vi "Wyznaczenie odległości robota od sartu na podstawie współrzędnych.vi"(7 "Azymut robota\n pocz/nowy":dbl caption="Azymut robota pocz/nowy" min=0.0 max=360.0, 10 "Parametry odwzorowania Ziemi (WGS84)":cluster{"a":dbl, "b":dbl}={"a"=6378137.0, "b"=6356752.3142} {"b" format="%#.6g"; "a" format="%#.6g"}, 11 "Pocz. poł.":T1 {"UTM"."N [m]" format="%#_10g"}) -> (0 "error out":errorcluster, 2 "Rzeczywista odległość robota od startu [m]":cluster{"X [m]":dbl, "Y [m]":dbl}, 3 "Aktualne położenie":T2 {"Szerokośc geograficzna - GPS" format="%_9f"; "Długość geograficzna - GPS" format="%_9f"; "Położenie \nrobota  UTM"."E [m]" format="%#_10g"; "Położenie \nrobota  UTM"."N [m]" format="%#_12g"})   [LabVIEW 2015, in "Biblioteka moduł map v3.lvlib" / "Pomocnicze.lvlib"]
doc: "Zadaniem pliku jest wyznaczenie odległości robota od punktu startowego na podstawie znanych współrzędnych geograficznych pliku startowego oraz odczytów z odbiornika GPS."
uses:
  Pomocnicze.lvlib
  Matematyczne/Matematyczne.lvlib
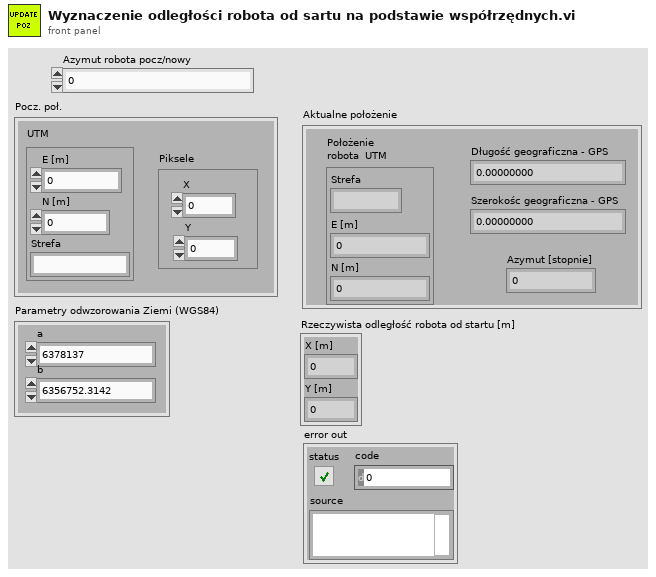
[diagram p1: front panel]
types:
  T1 = cluster{"UTM":cluster{"E [m]":dbl, "N [m]":dbl, "Strefa":string}, "Piksele":cluster{"X":i32, "Y":i32}}
  T2 = cluster{"Położenie \nrobota  UTM":cluster{"E [m]":ext, "N [m]":ext, "Strefa":string}, "Długość geograficzna - GPS":dbl, "Szerokośc geograficzna - GPS":dbl, "Azymut [stopnie]":dbl}
  T3 = cluster{"E [m]":ext, "N [m]":ext, "Strefa":string}
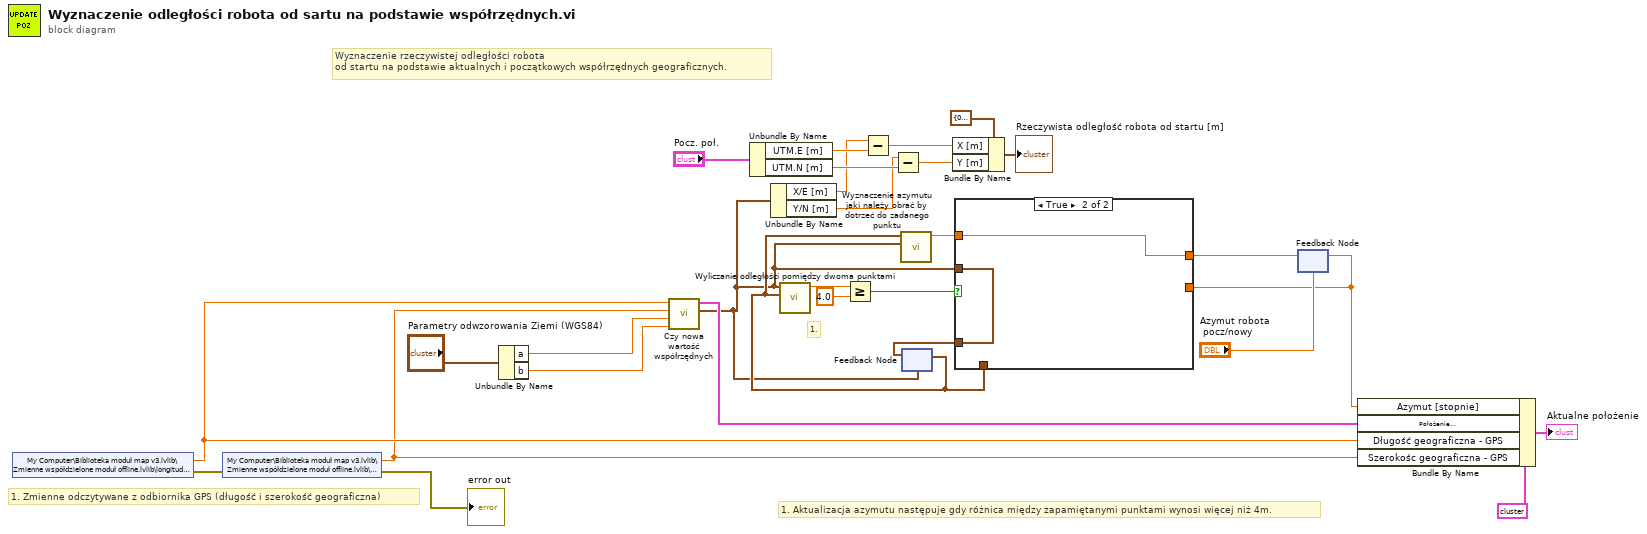
[diagram p0: block diagram]
diagram:
  # "1. Aktualizacja azymutu następuje gdy różnica między zapamiętanymi punktami wynosi więcej niż 4m."
  # "1."
  # "Wyznaczenie rzeczywistej odległości robota \nod startu na podstawie aktualnych i początkowych współrzędnych geograficznych."
  # "1. Zmienne odczytywane z odbiornika GPS (długość i szerokość geograficzna)"
  n1 = shared-variable "My Computer\\Biblioteka moduł map v3.lvlib\\Zmienne współdzielone moduł offline.lvlib\\longitude.longitude (deg)"() -> (w22:dbl, error out=w25:errorcluster)  [unwired: 1 in]
  n2 = shared-variable "My Computer\\Biblioteka moduł map v3.lvlib\\Zmienne współdzielone moduł offline.lvlib\\latitude.latitude (deg)"(error in=w25) -> (w21:dbl, error out=→"error out":errorcluster)
  n3 = Unbundle By Name("Parametry odwzorowania Ziemi (WGS84)") -> ("a"=w27:dbl, "b"=w28:dbl)
  n4 = call "Czy nowa wartość współrzędnych.vi"("b"=w28, "a"=w27, "szerokość geograficzna"=w21, "Długość geograficzna"=w22) -> ("Położenie"=w3:cluster{"X/E [m]":dbl, "Y/N [m]":dbl}, "Położenie \nrobota  UTM"=w20:T3)  [unwired: 5 in, 1 out]
  n5 = Unbundle By Name("Pocz. poł.") -> ("UTM.E [m]"=w18:dbl, "UTM.N [m]"=w17:dbl)
  n6 = Unbundle By Name(w3) -> ("X/E [m]"=w16:dbl, "Y/N [m]"=w15:dbl)
  n7 = Subtract(x=w16, y=w18) -> (x-y=w6:dbl)
  n8 = Subtract(x=w15, y=w17) -> (x-y=w5:dbl)
  n9 = feedback #1(w3) -> (w4:cluster{"X/E [m]":dbl, "Y/N [m]":dbl})
  n10 = call "Wyliczanie odległości pomiędzy dwoma punktami.vi"("Polozenie 1"=w4, "Polozenie in"=w3) -> ("Numeric"=w14:dbl)  [unwired: 9 in]
  n11 = Greater Or Equal?(x=w14, y=4.0) -> (x >= y?=w12:bool)
  n12 = call "Wyznaczenie azymutu jaki należy obrać by dotrzeć do zadanego punktu.vi"("Położenie końcowe"=w3, "Położenie aktualne"=w4) -> ("Azymut"=w11:dbl)  [unwired: 9 in]
  n13 = Bundle By Name(cluster=cluster{"X [m]":dbl, "Y [m]":dbl} {"X [m]"=0.0, "Y [m]"=0.0} ("event data"), "X [m]"=w6, "Y [m]"=w5) -> (→"Rzeczywista odległość robota od startu [m]":cluster{"X [m]":dbl, "Y [m]":dbl})
  n14 = feedback #2("Azymut robota\n pocz/nowy") -> (w1:dbl)
  n15 = case shown="True" w12 {
    tunnel: [w30 w33] -> w10
    tunnel: w11 -> [_ w33]
    tunnel: [w31 w32] -> w9
    tunnel: w3 -> [_ w32]
    tunnel: w4 -> [w31 _]
    tunnel: w1 -> [w30 _]
    frame False {
    }
    frame True {
    }
  }
  n16 = feedback-in #1(w9) -> ()
  n17 = feedback-in #2(w10) -> ()
  n18 = Bundle By Name(cluster=T2 {"Położenie \nrobota  UTM"={"E [m]"=0.0, "N [m]"=0.0, "Strefa"=""}, "Długość geograficzna - GPS"=0.0, "Szerokośc geograficzna - GPS"=0.0, "Azymut [stopnie]"=0.0} ("Aktualne położenie"), "Azymut [stopnie]"=w1, "Położenie \nrobota  UTM"=w20, "Długość geograficzna - GPS"=w22, "Szerokośc geograficzna - GPS"=w21) -> (→"Aktualne położenie":T2)
